vi "BallShear_BallSelection.vi"(8 "Selected Balls":dbl[][](array[numeric]), 11 "Check":bool) -> (3 "Ready":bool)   [LabVIEW 2013]
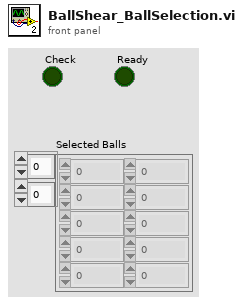
[diagram p1: front panel]
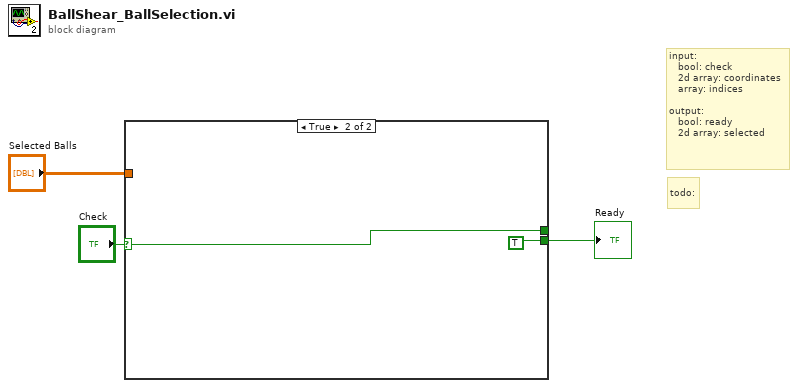
[diagram p0: block diagram]
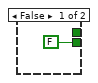
[diagram p2: hidden frame]
diagram:
  # "input:\n   bool: check\n   2d array: coordinates\n   array: indices\n\noutput: \n   bool: ready\n   2d array: selected"
  # "todo:"
  n1 = case shown="True" "Check" {
    tunnel: "Check" -> [_ _]
    tunnel: [FALSE ("Power") TRUE ("Power")] -> w2
    tunnel: "Selected Balls" -> [_ _]
    frame False {
    }
    frame True {
    }
  }
  "Ready" <- w2
